vi "CC Observation Generate Focus Move Step.vi"(8 "error in (no error)":errorcluster, 10 "Position":i32, 11 "Motor":i32) -> (0 "error out":errorcluster, 3 "Exp Step":T1={"Action"=enum."Acquire Images", "Data"=variant})   [LabVIEW 2024]
uses:
  typedefs/CC Script Step.ctl
  typedefs/CC enum Script Action.ctl
  Focus/Focus cluster MoveFocus Command Parameters.ctl
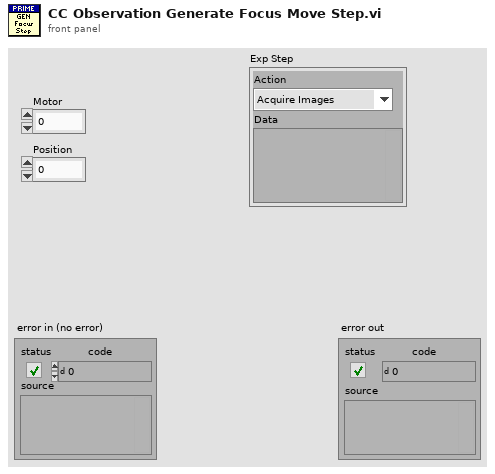
[diagram p1: front panel]
types:
  T1 = typedef "CC Script Step.ctl" = cluster{"Action":T2, "Data":variant}
  T2 = typedef "CC enum Script Action.ctl" = enum16{"Noop", "Define Object", "Define Exposure", "Define Dithering", "Acquire Images", "Set Filter Wheel", "Telescope Home", "Telescope Move", "Telescope RA DEC", "Focus Move Relative", "Focus Move Absolute", "Focus Set Home", "Macro", "Pause", "Ask User", "Define Random Dither", "CmdLine", "Outlet"}
  T3 = typedef "Focus cluster MoveFocus Command Parameters.ctl" = cluster{"Motor":i32, "Position":i32}
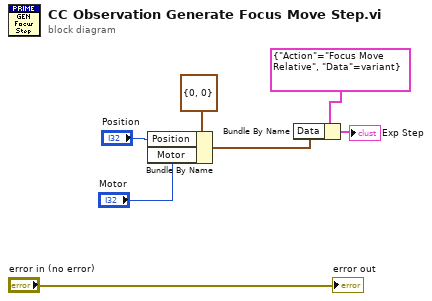
[diagram p0: block diagram]
diagram:
  n1 = Bundle By Name(cluster=T3 {"Motor"=0, "Position"=0} ("Cluster"), "Position"="Position", "Motor"="Motor") -> (w6:T3)
  n2 = Bundle By Name(cluster=T1 {"Action"=enum."Focus Move Relative", "Data"=variant} ("Cluster"), "Data"=w6) -> (→"Exp Step":T1)
  "error out" <- "error in (no error)"
